vi "总磷总氮测量数据储存.vi"   [LabVIEW 2016, in "斯坦道仪器.lvlib"]
types:
  T1 = cluster{"时间标识":timestamp, "监测值":sgl, "单位":u16, "数据标识":string, "因子编码":u32, "标样参考值":sgl, "F0":sgl, "F1":sgl, "F2":sgl, "F3":sgl, "F4":sgl, "F5":sgl, "F6":sgl, "F7":sgl, "X":sgl, "温度":sgl, "湿度":sgl, "量程标识":string}
  T2 = enum16{"维护数据", "水样测试", "标样核查", "零点核查", "跨度核查", "空白测试", "平行样测试", "加标回收", "空白校准", "标样校准", "初始化（清洗）"}
  T3 = cluster{"系统时间":timestamp, "工作状态":enum16{"空闲", "水样测试", "标样核查", "零点核查", "跨度核查", "空白测试", "平行样测试", "加标回收", "空白校准", "标样校准", "初始化（清洗）"}, "测量模式":enum16{"待机", "连续模式", "周期模式", "定点模式", "受控模式", "手动模式"}, "告警代码":enum16{"无告警", "缺试剂告警", "缺水样告警", "缺蒸馏水告警", "缺标液告警", "仪表漏液告警", "标定异常告警", "超量程告警", "加热异常", "低试剂预警", "超上限告警", "超下限告警", "仪表内部其他异常", "滴定异常告警", "电极异常告警", "量程切换告警", "参数设置告警", "PH电极电位异常", "电导率电极异常", "浊度光度异常", "溶解氧电极异常", "溶解氧光强异常", "温度异常告警", "PH异常告警", "溶解氧异常告警", "电导率异常告警", "浊度异常告警", "叶绿素异常告警", "藻密度异常告警", "蓝绿藻异常告警", "ORP异常告警", "氨氮异常告警", "清洁刷异常告警", "SD卡异常告警", "蓝牙异常告警", "Wifi异常告警", "流程异常告警"}, "故障代码":enum16{"无故障", "电机故障", "温度故障", "通讯故障", "滴定故障"}, "日志代码":u16, "软件版本":u16, "F0":sgl, "F1":sgl, "F2":sgl, "F3":sgl, "T":sgl, "H":sgl, "id":u16, "flowid":u16, "量程":u16, "总磷控温温度1":sgl, "营养盐控温温度2":sgl, "ADC":sgl}
  T4 = enum16{"空闲", "水样测试", "标样核查", "零点核查", "跨度核查", "空白测试", "平行样测试", "加标回收", "空白校准", "标样校准", "初始化（清洗）"}
  T5 = cluster{"因子编码":u32, "单位":u16, "标样参考值":sgl, "水样数据时间":timestamp, "水样实测值":sgl, "水样数据标识":string, "标样数据时间":timestamp, "标样实测值":sgl, "标样数据标识":string, "空白数据时间":timestamp, "空白实测值":sgl, "空白数据标识":string, "零点核查数据时间":timestamp, "零点核查实测值":sgl, "零点核查数据标识":string, "跨度核查数据时间":timestamp, "跨度核查实测值":sgl, "跨度核查数据标识":string, "加标回收数据时间":timestamp, "加标回收实测值":sgl, "加标回收数据标识":string, "平行样数据时间":timestamp, "平行样实测值":sgl, "平行样数据标识":string, "F0":sgl, "F1":sgl, "F2":sgl, "F3":sgl, "F4":sgl, "F5":sgl, "F6":sgl, "F7":sgl, "温度":sgl, "湿度":sgl, "X值":sgl}
  T6 = cluster{"总磷跨度值":dbl, "总磷零点标准液浓度":dbl, "总磷跨度标准液浓度":dbl, "总磷标准液标准浓度":dbl, "总氮跨度值":dbl, "总氮零点标准液浓度":dbl, "总氮跨度标准液浓度":dbl, "总氮标准液标准浓度":dbl}
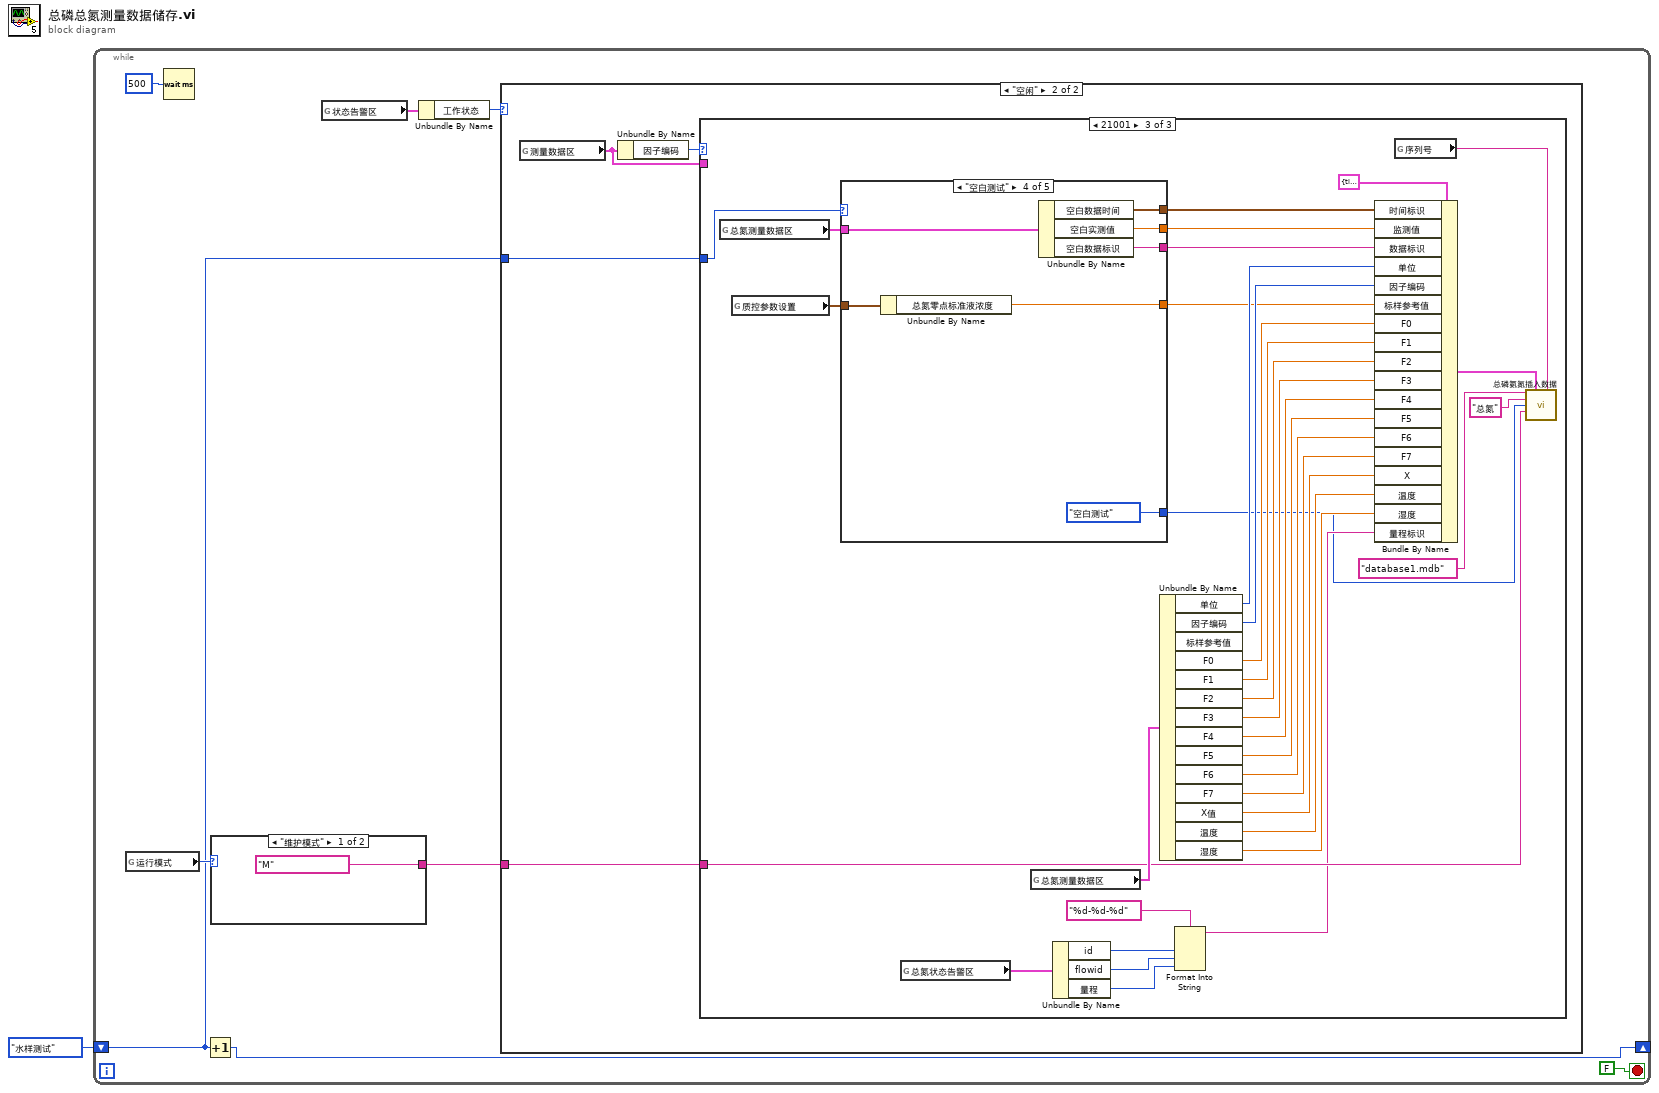
[diagram p0: block diagram]
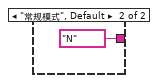
[diagram p2: hidden frame]
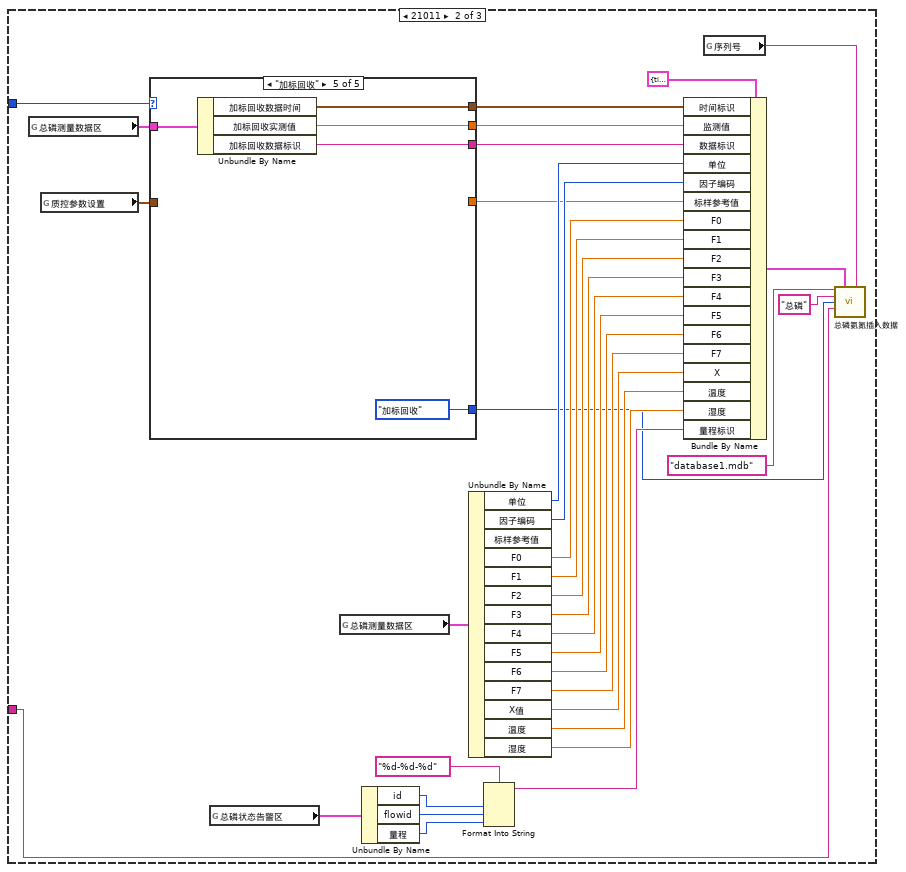
[diagram p5: hidden frame]
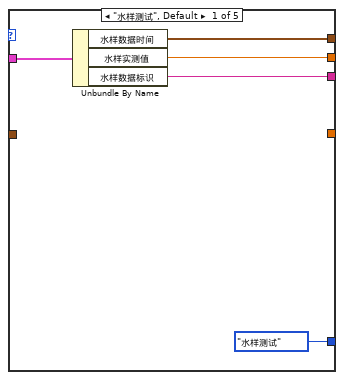
[diagram p6: hidden frame]
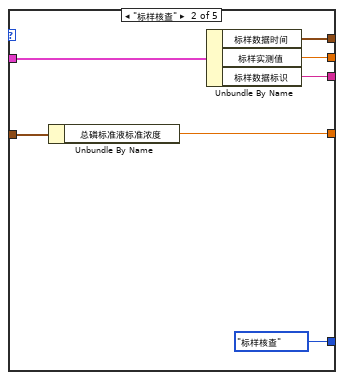
[diagram p7: hidden frame]
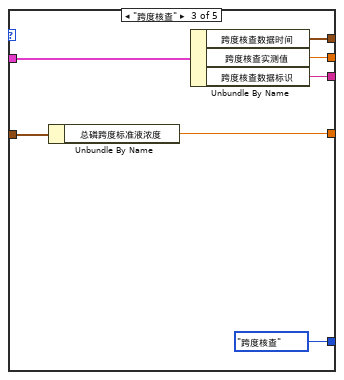
[diagram p8: hidden frame]
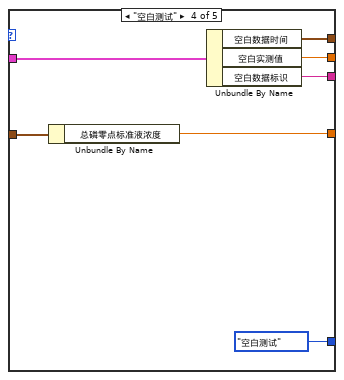
[diagram p9: hidden frame]
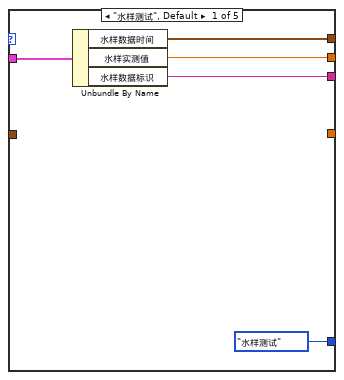
[diagram p10: hidden frame]
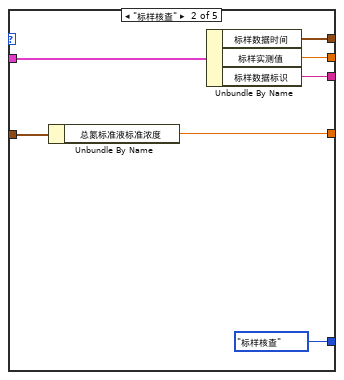
[diagram p11: hidden frame]
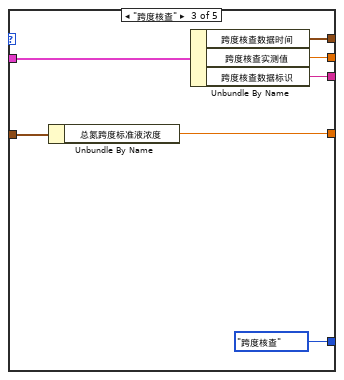
[diagram p12: hidden frame]
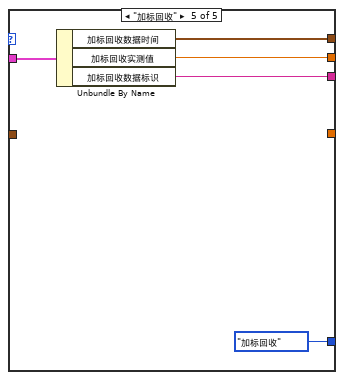
[diagram p13: hidden frame]
diagram:
  n1 = while {
    shift-right: [w4] -> _
    shift-left: enum16{"水样测试", "标样核查", "跨度核查", "空白测试", "加标回收"}."水样测试" ("测量模式") -> [w3]
    stop <- FALSE stop-if-true
    n2 = global read "系统变量.vi" "运行模式"() -> (w6:enum16{"维护模式", "常规模式", "应急模式", "质控模式"})
    n3 = Wait (ms)(milliseconds to wait=u32 500 ("等待时间（毫秒）")) -> ()  [unwired: 1 out]
    n4 = Increment(x=w3) -> (x+1=w4:enum16{"水样测试", "标样核查", "跨度核查", "空白测试", "加标回收"})
    n5 = case shown="\"维护模式\"" w6 {
      tunnel: ["M" ("数据标记表") "N" ("数据标记表")] -> w5
      frame "维护模式" {
      }
      frame "常规模式", Default {
      }
    }
    n6 = global read "VAR总磷总氮全局变量.vi" "状态告警区"() -> (w2:T3)
    n7 = Unbundle By Name(w2) -> ("工作状态"=w7:T4)
    n8 = case shown="\"空闲\"" w7 {
      tunnel: w5 -> [_ w13]
      tunnel: w3 -> [_ w12]
      frame Default {
      }
      frame "空闲" {
        n9 = global read "VAR总磷总氮全局变量.vi" "测量数据区"() -> (w15:T5)
        n10 = Unbundle By Name(w15) -> ("因子编码"=w14:u32)
        n11 = case shown="21001" w14 {
          tunnel: w15 -> [_ _ _]
          tunnel: w13 -> [_ w20 w103]
          tunnel: w12 -> [_ w19 w88]
          frame Default {
          }
          frame 21011 {
            n12 = global read "VAR总磷总氮全局变量.vi" "总磷测量数据区"() -> (w48:T5)
            n13 = global read "总磷总氮断电保存全局变量.vi" "质控参数设置"() -> (w17:T6)
            n14 = case shown="\"加标回收\"" w19 {
              tunnel: w48 -> [w54 w61 w68 w75 w80]
              tunnel: [w53 w60 w67 w74 w79] -> w24
              tunnel: [w52 w59 w66 w73 w78] -> w25
              tunnel: [w51 w58 w65 w72 w77] -> w26
              tunnel: [T2."水样测试" ("测量模式") T2."标样核查" ("测量模式") T2."跨度核查" ("测量模式") T2."空白测试" ("测量模式") T2."加标回收" ("测量模式")] -> w23
              tunnel: w17 -> [_ w56 w63 w70 _]
              tunnel: [_ w55 w62 w69 _] -> w16
              frame "水样测试", Default {
                n15 = Unbundle By Name(w54) -> ("水样数据时间"=w53:timestamp, "水样实测值"=w52:sgl, "水样数据标识"=w51:string)
              }
              frame "标样核查" {
                n16 = Unbundle By Name(w56) -> ("总磷标准液标准浓度"=w55:dbl)
                n17 = Unbundle By Name(w61) -> ("标样数据时间"=w60:timestamp, "标样实测值"=w59:sgl, "标样数据标识"=w58:string)
              }
              frame "跨度核查" {
                n18 = Unbundle By Name(w63) -> ("总磷跨度标准液浓度"=w62:dbl)
                n19 = Unbundle By Name(w68) -> ("跨度核查数据时间"=w67:timestamp, "跨度核查实测值"=w66:sgl, "跨度核查数据标识"=w65:string)
              }
              frame "空白测试" {
                n20 = Unbundle By Name(w70) -> ("总磷零点标准液浓度"=w69:dbl)
                n21 = Unbundle By Name(w75) -> ("空白数据时间"=w74:timestamp, "空白实测值"=w73:sgl, "空白数据标识"=w72:string)
              }
              frame "加标回收" {
                n22 = Unbundle By Name(w80) -> ("加标回收数据时间"=w79:timestamp, "加标回收实测值"=w78:sgl, "加标回收数据标识"=w77:string)
              }
            }
            n23 = global read "VAR总磷总氮全局变量.vi" "总磷状态告警区"() -> (w18:T3)
            n24 = global read "VAR总磷总氮全局变量.vi" "总磷测量数据区"() -> (w31:T5)
            n25 = Unbundle By Name(w18) -> ("id"=w49:u16, "flowid"=w33:u16, "量程"=w32:u16)
            n26 = Unbundle By Name(w31) -> ("单位"=w47:u16, "因子编码"=w46:u32, "F0"=w45:sgl, "F1"=w44:sgl, "F2"=w43:sgl, "F3"=w42:sgl, "F4"=w41:sgl, "F5"=w40:sgl, "F6"=w39:sgl, "F7"=w38:sgl, "X值"=w37:sgl, "温度"=w36:sgl, "湿度"=w35:sgl)  [unwired: 1 out]
            n27 = Format Into String(format string="%d-%d-%d" ("格式字符串"), w49, w33, w32) -> (resulting string=w34:string)  [unwired: 2 in, 1 out]
            n28 = Bundle By Name(cluster=T1 {"时间标识"=timestamp(0 s since 1904-01-01), "监测值"=0.0, "单位"=0, "数据标识"="", "因子编码"=0, "标样参考值"=0.0, "F0"=0.0, "F1"=0.0, "F2"=0.0, "F3"=0.0, "F4"=0.0, "F5"=0.0, "F6"=0.0, "F7"=0.0, "X"=0.0, "温度"=0.0, "湿度"=0.0, "量程标识"=""} ("data"), "时间标识"=w24, "监测值"=w25, "数据标识"=w26, "单位"=w47, "因子编码"=w46, "标样参考值"=w16, "F0"=w45, "F1"=w44, "F2"=w43, "F3"=w42, "F4"=w41, "F5"=w40, "F6"=w39, "F7"=w38, "X"=w37, "温度"=w36, "湿度"=w35, "量程标识"=w34) -> (w28:T1)
            n29 = global read "VAR总磷总氮全局变量.vi" "序列号"() -> (w27:string)
            n30 = call "总磷氨氮插入数据.vi"("database"="database1.mdb", "data"=w28, "SN"=w27, "table"="总磷", "测量模式"=w23, "数据标记表"=w20) -> ()  [unwired: 9 in, 1 out]
          }
          frame 21001 {
            n31 = global read "VAR总磷总氮全局变量.vi" "总氮测量数据区"() -> (w87:T5)
            n32 = global read "总磷总氮断电保存全局变量.vi" "质控参数设置"() -> (w82:T6)
            n33 = case shown="\"空白测试\"" w88 {
              tunnel: w87 -> [w119 w126 w133 w140 w145]
              tunnel: [w118 w125 w132 w139 w144] -> w86
              tunnel: [w117 w124 w131 w138 w143] -> w85
              tunnel: [w116 w123 w130 w137 w142] -> w84
              tunnel: [T2."水样测试" ("测量模式") T2."标样核查" ("测量模式") T2."跨度核查" ("测量模式") T2."空白测试" ("测量模式") T2."加标回收" ("测量模式")] -> w83
              tunnel: w82 -> [_ w121 w128 w135 _]
              tunnel: [_ w120 w127 w134 _] -> w81
              frame "水样测试", Default {
                n34 = Unbundle By Name(w119) -> ("水样数据时间"=w118:timestamp, "水样实测值"=w117:sgl, "水样数据标识"=w116:string)
              }
              frame "标样核查" {
                n35 = Unbundle By Name(w121) -> ("总氮标准液标准浓度"=w120:dbl)
                n36 = Unbundle By Name(w126) -> ("标样数据时间"=w125:timestamp, "标样实测值"=w124:sgl, "标样数据标识"=w123:string)
              }
              frame "跨度核查" {
                n37 = Unbundle By Name(w128) -> ("总氮跨度标准液浓度"=w127:dbl)
                n38 = Unbundle By Name(w133) -> ("跨度核查数据时间"=w132:timestamp, "跨度核查实测值"=w131:sgl, "跨度核查数据标识"=w130:string)
              }
              frame "空白测试" {
                n39 = Unbundle By Name(w135) -> ("总氮零点标准液浓度"=w134:dbl)
                n40 = Unbundle By Name(w140) -> ("空白数据时间"=w139:timestamp, "空白实测值"=w138:sgl, "空白数据标识"=w137:string)
              }
              frame "加标回收" {
                n41 = Unbundle By Name(w145) -> ("加标回收数据时间"=w144:timestamp, "加标回收实测值"=w143:sgl, "加标回收数据标识"=w142:string)
              }
            }
            n42 = global read "VAR总磷总氮全局变量.vi" "总氮状态告警区"() -> (w111:T3)
            n43 = global read "VAR总磷总氮全局变量.vi" "总氮测量数据区"() -> (w114:T5)
            n44 = Unbundle By Name(w111) -> ("id"=w107:u16, "flowid"=w106:u16, "量程"=w105:u16)
            n45 = Unbundle By Name(w114) -> ("单位"=w113:u16, "因子编码"=w112:u32, "F0"=w101:sgl, "F1"=w100:sgl, "F2"=w99:sgl, "F3"=w98:sgl, "F4"=w97:sgl, "F5"=w96:sgl, "F6"=w95:sgl, "F7"=w94:sgl, "X值"=w93:sgl, "温度"=w92:sgl, "湿度"=w91:sgl)  [unwired: 1 out]
            n46 = Format Into String(format string="%d-%d-%d" ("格式字符串"), w107, w106, w105) -> (resulting string=w90:string)  [unwired: 2 in, 1 out]
            n47 = Bundle By Name(cluster=T1 {"时间标识"=timestamp(0 s since 1904-01-01), "监测值"=0.0, "单位"=0, "数据标识"="", "因子编码"=0, "标样参考值"=0.0, "F0"=0.0, "F1"=0.0, "F2"=0.0, "F3"=0.0, "F4"=0.0, "F5"=0.0, "F6"=0.0, "F7"=0.0, "X"=0.0, "温度"=0.0, "湿度"=0.0, "量程标识"=""} ("data"), "时间标识"=w86, "监测值"=w85, "数据标识"=w84, "单位"=w113, "因子编码"=w112, "标样参考值"=w81, "F0"=w101, "F1"=w100, "F2"=w99, "F3"=w98, "F4"=w97, "F5"=w96, "F6"=w95, "F7"=w94, "X"=w93, "温度"=w92, "湿度"=w91, "量程标识"=w90) -> (w89:T1)
            n48 = global read "VAR总磷总氮全局变量.vi" "序列号"() -> (w104:string)
            n49 = call "总磷氨氮插入数据.vi"("database"="database1.mdb", "data"=w89, "SN"=w104, "table"="总氮", "测量模式"=w83, "数据标记表"=w103) -> ()  [unwired: 9 in, 1 out]
          }
        }
      }
    }
  }
